vi "Get Pattern.vi"(11 "Reflective Memory File in":refnum<class "Reflective Memory File.lvclass">) -> (2 "file extension":string)   [LabVIEW 2015, in "RefMem DMA Custom Device.lvlib" / "Reflective Memory File.lvclass"]
uses:
  Reflective Memory File.lvclass
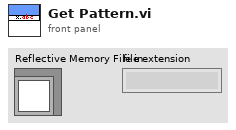
[diagram p1: front panel]
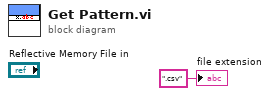
[diagram p0: block diagram]
diagram:
  "file extension" <- ".csv" ("file extension")
